vi "Project Local Root Directory.vi"() -> (3 "Code root's folder":path)   [LabVIEW 2018, in "Personalities Tool.lvlib"]
doc: "This VI gets the project's root directory for easy path creation from both the EXE and the development environment."
uses:
  Personalities Tool.lvlib
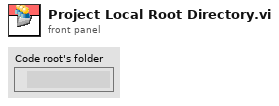
[diagram p1: front panel]
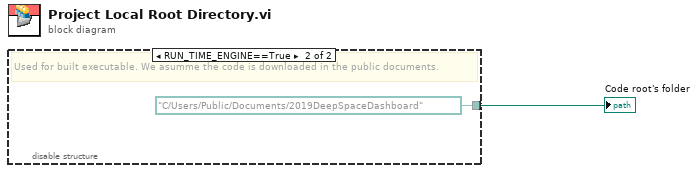
[diagram p0: block diagram]
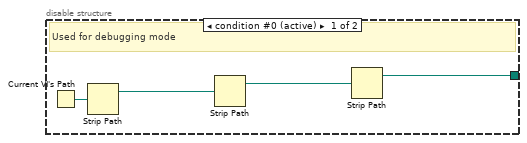
[diagram p2: hidden frame]
diagram:
  n1 = disable-structure shown="RUN_TIME_ENGINE==True" {
    disable-tunnel: [w5 path "C:/Users/Public/Documents/2019DeepSpaceDashboard" ("stripped path")] -> w1
    frame condition #0 (active) {
      # "Used for debugging mode"
      n2 = Current VI's Path() -> (path=w4:path)
      n3 = Strip Path(path=w4) -> (stripped path=w3:path)  [unwired: 1 out]
      n4 = Strip Path(path=w3) -> (stripped path=w2:path)  [unwired: 1 out]
      n5 = Strip Path(path=w2) -> (stripped path=w5:path)  [unwired: 1 out]
    }
    frame condition #1 {
      # "Used for built executable. We asumme the code is downloaded in the public documents."
    }
  }
  "Code root's folder" <- w1
